vi "Timeperdivknob.vi"(0 "Dial":u32(knob) scale=0.0..44.0, 3 "error in (no error)":errorcluster) -> (5 "Time/Div.":dbl format="%.2e", 8 "error out":errorcluster)   [LabVIEW 2014]
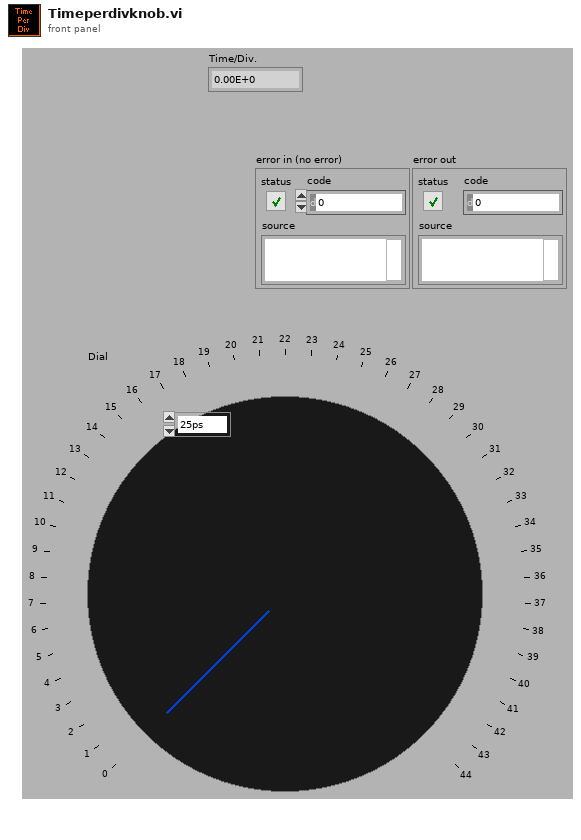
[diagram p1: front panel]
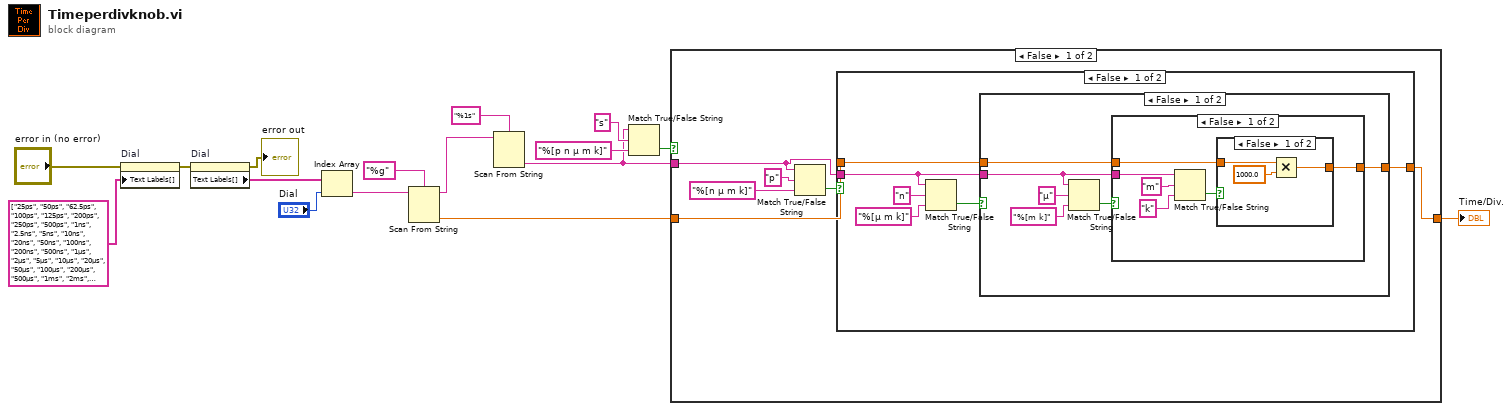
[diagram p0: block diagram]
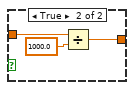
[diagram p2: hidden frame]
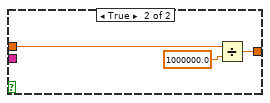
[diagram p3: hidden frame]
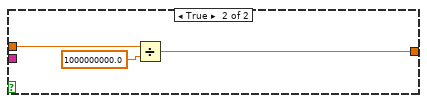
[diagram p4: hidden frame]
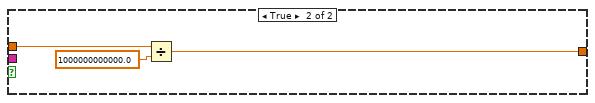
[diagram p5: hidden frame]
diagram:
  n1 = property on="Dial" class="Knob (strict)"(error in="error in (no error)", "Text Labels[]"=string[] ["25ps", "50ps", "62.5ps", "100ps", "125ps", "200ps", "250ps", "500ps", "1ns", "2.5ns", "5ns", "10ns", "20ns", "50ns", "100ns", "200ns", "500ns", "1µs", "2µs", "5µs", "10µs", "20µs", "50µs", "100µs", "200µs", "500µs", "1ms", "2ms", "5ms", "10ms", "20ms", "50ms", "100ms", "200ms", "500ms", "1s", "2s", "5s", "10s", "20s", "50s", "100s", "200s", "500s", "1ks"]) -> (error out=w12:errorcluster)  [unwired: 1 in, 1 out]
  n2 = property on="Dial" class="Knob (strict)"(error in=w12) -> (error out=→"error out":errorcluster, "Text Labels[]"=w13:string[])  [unwired: 1 in, 1 out]
  n3 = Index Array(array=w13, index="Dial") -> (element=w1:string)
  n4 = Scan From String(format string="%g", input string=w1) -> (remaining string=w10:string, output 1=w4:dbl)  [unwired: 3 in, 2 out]
  n5 = Scan From String(format string="%1s", input string=w10) -> (output 1=w3:string)  [unwired: 3 in, 3 out]
  n6 = Match True/False String(2:"%[p n µ m k]" ("false string"), 3:"s" ("true string"), 4:w3) -> (0:w7:bool)  [unwired: 1 out]
  n7 = case shown="False" w7 {
    tunnel: w4 -> [w19 w56]
    tunnel: [w17 w56] -> w2
    tunnel: w3 -> [w18 _]
    frame False {
      n8 = Match True/False String(2:"%[n µ m k]" ("false string"), 3:"p" ("true string"), 4:w18) -> (0:w21:bool)  [unwired: 1 out]
      n9 = case shown="False" w21 {
        tunnel: w19 -> [w25 w55]
        tunnel: [w24 w53] -> w17
        tunnel: w18 -> [w23 _]
        frame False {
          n10 = Match True/False String(2:"%[µ m k]" ("false string"), 3:"n" ("true string"), 4:w23) -> (0:w28:bool)  [unwired: 1 out]
          n11 = case shown="False" w28 {
            tunnel: w25 -> [w31 w52]
            tunnel: [w30 w50] -> w24
            tunnel: w23 -> [w29 _]
            frame False {
              n12 = Match True/False String(2:"%[m k]" ("false string"), 3:"µ" ("true string"), 4:w29) -> (0:w34:bool)  [unwired: 1 out]
              n13 = case shown="False" w34 {
                tunnel: w31 -> [w36 w49]
                tunnel: [w35 w47] -> w30
                tunnel: w29 -> [w40 _]
                frame False {
                  n14 = Match True/False String(2:"k" ("false string"), 3:"m" ("true string"), 4:w40) -> (0:w37:bool)  [unwired: 1 out]
                  n15 = case shown="False" w37 {
                    tunnel: w36 -> [w43 w46]
                    tunnel: [w41 w44] -> w35
                    frame False {
                      n16 = Multiply(x=w43, y=1000.0) -> (x*y=w41:dbl)
                    }
                    frame True {
                      n17 = Divide(x=w46, y=1000.0) -> (x/y=w44:dbl)
                    }
                  }
                }
                frame True {
                  n18 = Divide(x=w49, y=1000000.0) -> (x/y=w47:dbl)
                }
              }
            }
            frame True {
              n19 = Divide(x=w52, y=1000000000.0) -> (x/y=w50:dbl)
            }
          }
        }
        frame True {
          n20 = Divide(x=w55, y=1000000000000.0) -> (x/y=w53:dbl)
        }
      }
    }
    frame True {
    }
  }
  "Time/Div." <- w2
